vi "Set Function.vi"(7 "State":enum16{"Set", "Get"}(ring)=enum."Get", 8 "error in (no error)":errorcluster, 10 "Action":T1) -> (0 "error out":errorcluster, 2 "Get Action":T1)   [LabVIEW 2019]
uses:
  controls/Set_Function.ctl
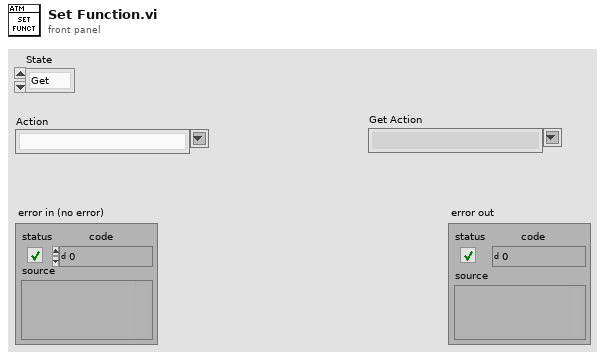
[diagram p1: front panel]
types:
  T1 = typedef "Set_Function.ctl" = string
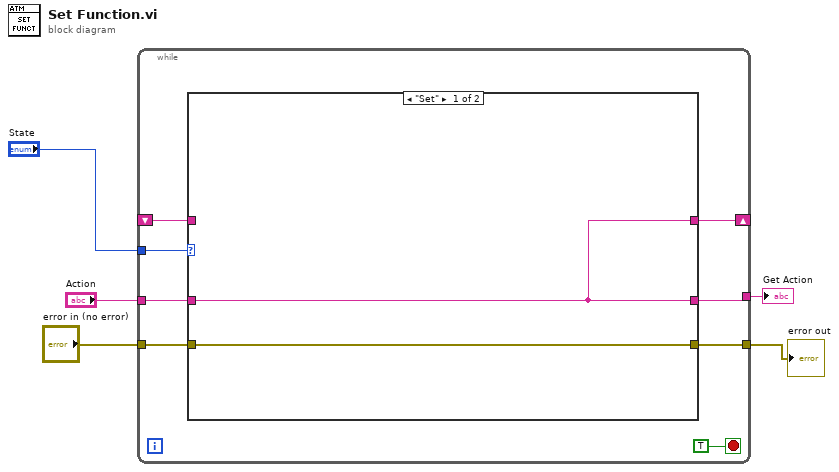
[diagram p0: block diagram]
diagram:
  n1 = while {
    tunnel: "State" -> [w13]
    tunnel: "Action" -> [w12]
    shift-right: [w11] -> _
    shift-left: _ -> [w9]
    tunnel: [w10] -> w3
    tunnel: "error in (no error)" -> [w7]
    tunnel: [w6] -> w1
    stop <- TRUE stop-if-true
    n2 = case shown="\"Set\"" w13 {
      tunnel: w12 -> [w15 _]
      tunnel: [w15 w17] -> w11
      tunnel: [w15 w17] -> w10
      tunnel: w9 -> [_ w17]
      tunnel: w7 -> [w14 w16]
      tunnel: [w14 w16] -> w6
      frame "Set" {
      }
      frame "Get", Default {
      }
    }
  }
  "Get Action" <- w3
  "error out" <- w1
